vi "Encoder.vi"(0 "Relative_Motor_position":dbl) -> (1 "Pulse_duration":u32, 2 "Pulse_duration_cent":u32, 3 "recommended delay":dbl)   [LabVIEW 2018]
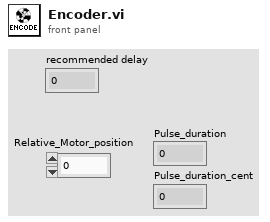
[diagram p1: front panel]
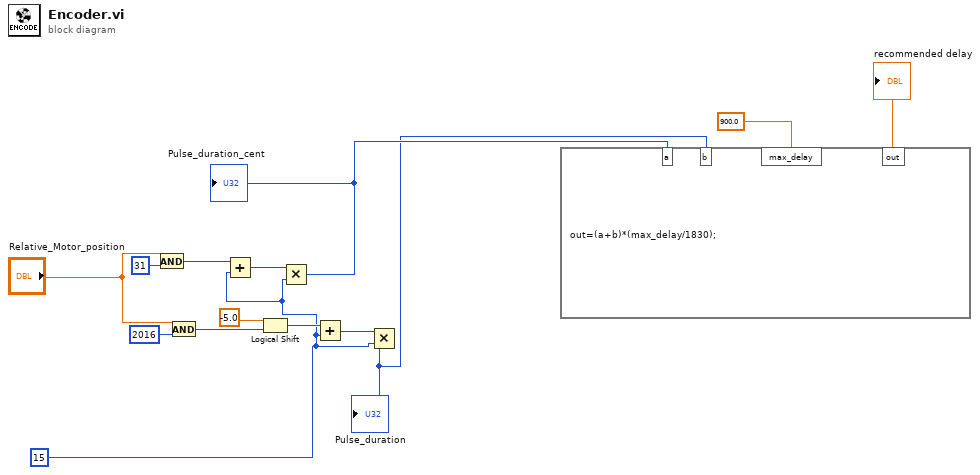
[diagram p0: block diagram]
diagram:
  w5 = 15 ("y")
  n1 = And(x="Relative_Motor_position", y=u32 31 ("x")) -> (x .and. y?=w9:i32)
  n2 = And(x="Relative_Motor_position", y=u32 2016 ("x")) -> (x .and. y?=w11:i32)
  n3 = Add(x=w9, y=w5) -> (x+y=w8:i32)
  n4 = Logical Shift(y=-5.0 ("x"), x=w11) -> (x << y=w6:i32)
  n5 = Multiply(x=w8, y=w5) -> (x*y=w4:i32)
  "Pulse_duration_cent" <- w4
  n6 = Add(x=w6, y=w5) -> (x+y=w7:i32)
  n7 = Multiply(x=w7, y=w5) -> (x*y=w3:i32)
  "Pulse_duration" <- w3
  n8 = formula code="out=(a+b)*(max_delay/1830);"("a"=w4, "b"=w3, "max_delay"=900.0 ("input variable")) -> ("out"=→"recommended delay":dbl)
